vi "SQL_EDITOR_records_click_discard.vi"(9 "uneditable_columns":string[](array[string]), 10 "CellPosition":T2, 11 "event_structure_shift_register_in":T1={"REF_EDIT_clicked_row"=-1, "REF_EDIT_selected_row"=-1, "SQL_EDIT_clicked_row"=-1, "SQL_EDIT_selected_row"=-1, "ARCH_EDIT_selected_row"=-1, "ARCH_EDIT_clicked_row"=-1, "USER_EDIT_selected_row"=-1, "USER_EDIT_clicked_row"=-1, "REPORT_GEAR_toggle_all_results"=FALSE}) -> (2 "Discard?":bool, 3 "event_structure_shift_register_out":T1={"REF_EDIT_clicked_row"=-1, "REF_EDIT_selected_row"=-1, "SQL_EDIT_clicked_row"=-1, "SQL_EDIT_selected_row"=-1, "ARCH_EDIT_selected_row"=-1, "ARCH_EDIT_clicked_row"=-1, "USER_EDIT_selected_row"=-1, "USER_EDIT_clicked_row"=-1, "REPORT_GEAR_toggle_all_results"=FALSE})   [LabVIEW 2019]
uses:
  CLIENT_event_structure_shift_register.ctl
  <vilib>/Utility/miscctls.llb/LVRowAndColumnTypeDef.ctl
  FGV/SQL_EDITOR_records_display/FGV_SQL_EDITOR_records_display.ctl
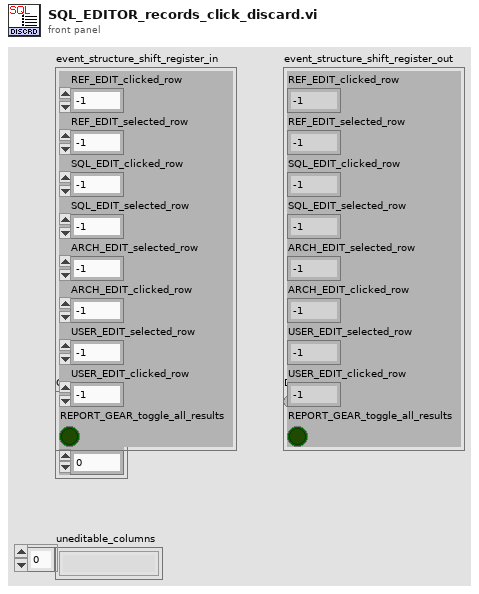
[diagram p1: front panel]
types:
  T1 = typedef "CLIENT_event_structure_shift_register.ctl" = cluster{"REF_EDIT_clicked_row":i32, "REF_EDIT_selected_row":i32, "SQL_EDIT_clicked_row":i32, "SQL_EDIT_selected_row":i32, "ARCH_EDIT_selected_row":i32, "ARCH_EDIT_clicked_row":i32, "USER_EDIT_selected_row":i32, "USER_EDIT_clicked_row":i32, "REPORT_GEAR_toggle_all_results":bool}
  T2 = typedef "LVRowAndColumnTypeDef.ctl" = cluster{"Row":i32, "Column":i32}
  T3 = typedef "FGV_SQL_EDITOR_records_display.ctl" = enum16{"initialize", "set_table_name", "set_column_name", "set_value_to_select", "set_order_by", "set_asc_desc", "set_headers", "set_records", "get_table_name", "get_column_name", "get_value_to_select", "get_headers", "get_all_info", "record_added?", "record_inserted?", "record_edited?", "record_updated?", "record_deleted?", "discard_changes"}
  T4 = typedef "SQL_EDITOR_all_info.ctl" = cluster{"table":string, "column":string, "value_to_select":string, "order_by":string, "asc_desc":string, "headers":string[], "uneditable_columns":string[], "uneditable_columns":i32[], "editable_columns":i32[], "values_in_database":string[][], "size":cluster{"columns":i32, "SQL_rows":i32, "disp_rows":i32}, "SQL_record_states":T5[]}
  T5 = typedef "SQL_record_states.ctl" = enum16{"Equal", "Added", "Edited", "Deleted"}
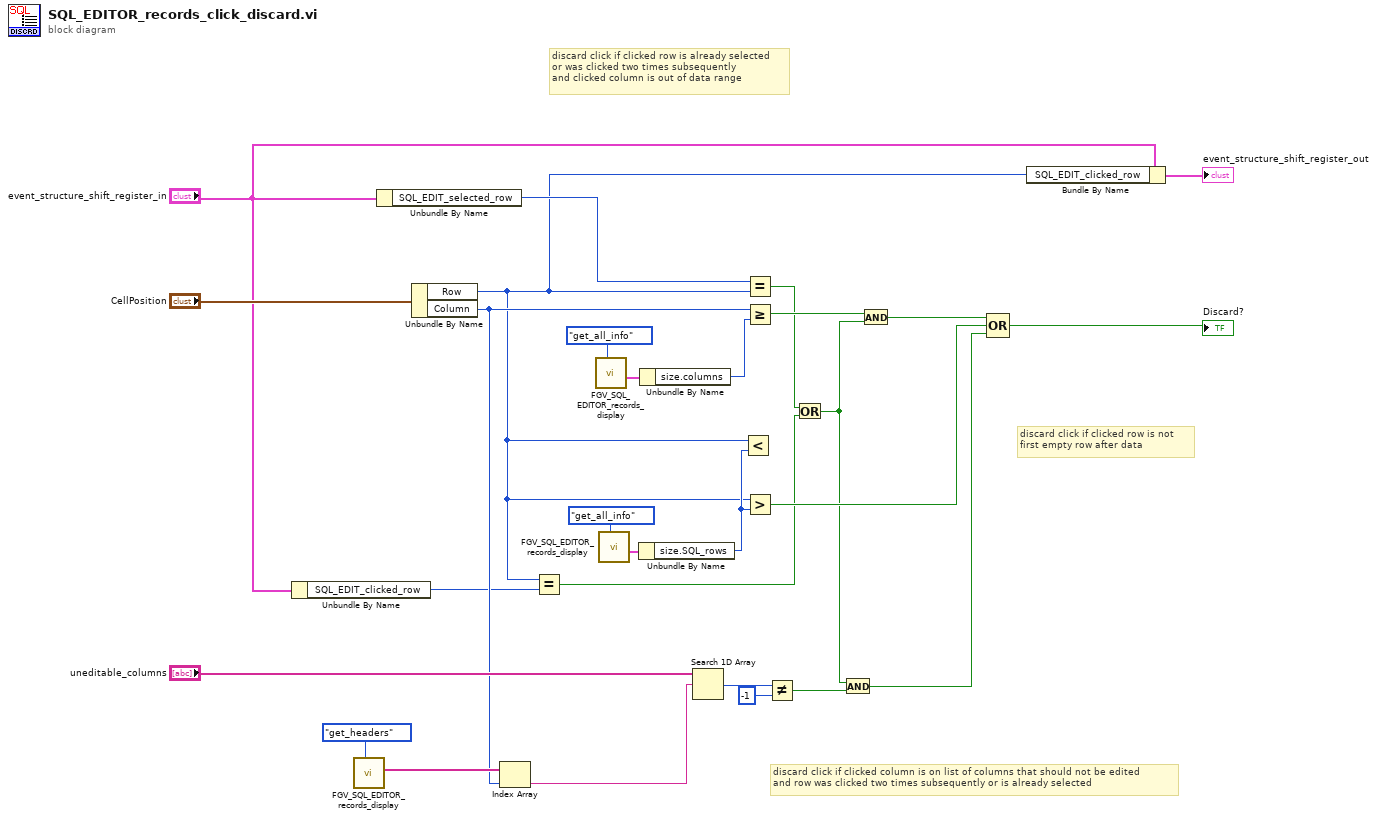
[diagram p0: block diagram]
diagram:
  # "discard click if clicked column is on list of columns that should not be edited\nand row was clicked two times subsequently or is already selected"
  # "discard click if clicked row is not \nfirst empty row after data"
  # "discard click if clicked row is already selected\nor was clicked two times subsequently\nand clicked column is out of data range"
  n1 = Unbundle By Name("event_structure_shift_register_in") -> ("SQL_EDIT_clicked_row"=w8:i32)
  n2 = call "FGV_SQL_EDITOR_records_display.vi"("options"=FGV_SQL_EDITOR_records_display."get_headers") -> ("array_param_output"=w22:string[])  [unwired: 7 in, 3 out]
  n3 = Unbundle By Name("event_structure_shift_register_in") -> ("SQL_EDIT_selected_row"=w13:i32)
  n4 = Unbundle By Name("CellPosition") -> ("Row"=w7:i32, "Column"=w21:i32)
  n5 = Index Array(array=w22, index=w21) -> (element=w20:string)
  n6 = Equal?(x=w7, y=w8) -> (x = y?=w4:bool)
  n7 = call "FGV_SQL_EDITOR_records_display.vi"("options"=FGV_SQL_EDITOR_records_display."get_all_info") -> ("all_info"=w2:T4)  [unwired: 7 in, 3 out]
  n8 = call "FGV_SQL_EDITOR_records_display.vi"("options"=FGV_SQL_EDITOR_records_display."get_all_info") -> ("all_info"=w1:T4)  [unwired: 7 in, 3 out]
  n9 = Unbundle By Name(w1) -> ("size.SQL_rows"=w11:i32)
  n10 = Unbundle By Name(w2) -> ("size.columns"=w25:i32)
  n11 = Search 1D Array(1D array="uneditable_columns", element=w20) -> (index of element=w19:i32)  [unwired: 1 in]
  n12 = Less?(x=w7, y=w11) -> ()  [unwired: 1 out]
  n13 = Equal?(x=w13, y=w7) -> (x = y?=w5:bool)
  n14 = Greater Or Equal?(x=w21, y=w25) -> (x >= y?=w6:bool)
  n15 = Greater?(x=w7, y=w11) -> (0:w14:bool)
  n16 = Not Equal?(x=w19, y=-1) -> (x != y?=w10:bool)
  n17 = Or(x=w5, y=w4) -> (x .or. y?=w3:bool)
  n18 = And(x=w3, y=w10) -> (x .and. y?=w16:bool)
  n19 = And(x=w6, y=w3) -> (x .and. y?=w17:bool)
  n20 = Compound Arithmetic op=OR(w17, w14, w16) -> (→"Discard?":bool)
  n21 = Bundle By Name(cluster="event_structure_shift_register_in", "SQL_EDIT_clicked_row"=w7) -> (→"event_structure_shift_register_out":T1)
